vi "datatype_conversion.vi"(10 "Data in":string) -> (2 "data":T1)   [LabVIEW 2020, in "configuration-data.lvclass"]
uses:
  configuration-data.lvclass
  value--cluster.ctl
  datatype--enum.ctl
  f3b64460-36c1-4435-9d0d-5d9a2c839281.vi
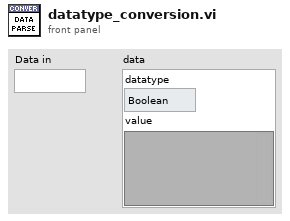
[diagram p1: front panel]
types:
  T1 = typedef "configuration-data.lvclass/value--cluster.ctl" = cluster{"datatype":T2, "value":variant}
  T2 = typedef "configuration-data.lvclass/datatype--enum.ctl" = enum16{"Boolean", "Double", "Integer", "String"}
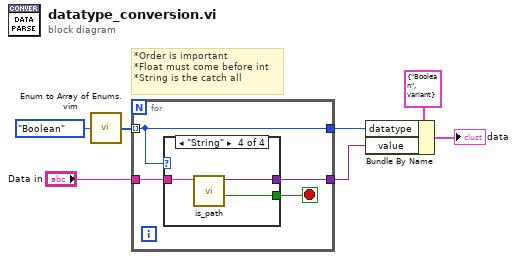
[diagram p0: block diagram]
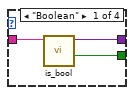
[diagram p2: hidden frame]
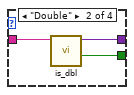
[diagram p3: hidden frame]
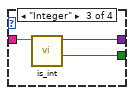
[diagram p4: hidden frame]
diagram:
  # "*Order is important\n*Float must come before int\n*String is the catch all"
  n1 = call "Enum to Array of Enums.vim"("enum"=datatype--enum."Boolean" ("datatype")) -> ("array of enums"=w6:T2[])
  n2 = for {
    tunnel: "Data in" -> [w11]
    tunnel: w6 -> [w8] mode=indexing
    tunnel: [w9] -> w4
    tunnel: [w8] -> w2
    stop <- w10 stop-if-true
    n3 = case shown="\"String\"" w8 {
      tunnel: w11 -> [w14 w17 w18 w23]
      tunnel: [w13 w15 w20 w21] -> w10
      tunnel: [w12 w16 w19 w22] -> w9
      frame "Boolean" {
        n4 = call "is_bool.vi"("data in"=w14) -> ("confirmed?"=w13:bool, "data out"=w12:variant)  [unwired: 9 in]
      }
      frame "Double" {
        n5 = call "is_dbl.vi"("data in"=w17) -> ("confirmed?"=w15:bool, "data out"=w16:variant)  [unwired: 9 in]
      }
      frame "Integer" {
        n6 = call "is_int.vi"("data in"=w18) -> ("confirmed?"=w20:bool, "data out"=w19:variant)  [unwired: 9 in]
      }
      frame "String" {
        n7 = call "is_path.vi"("data in"=w23) -> ("confirmed?"=w21:bool, "data out"=w22:variant)  [unwired: 9 in]
      }
    }
  }
  n8 = Bundle By Name(cluster=T1 {"datatype"=enum."Boolean", "value"=variant} ("data"), "datatype"=w2, "value"=w4) -> (→"data":T1)
